vi "NUM TO 2D LED (SubVI).vi"(1 "A":dbl) -> (0 "transposed array":bool[][](array[boolean]))   [LabVIEW 2019]
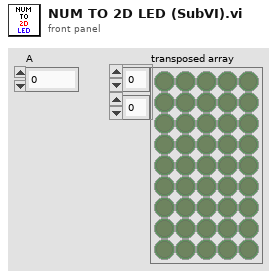
[diagram p1: front panel]
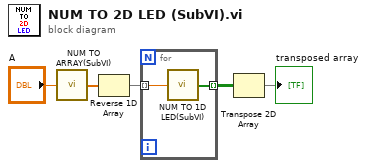
[diagram p0: block diagram]
diagram:
  n1 = call "NUM TO ARRAY(SubVI).vi"("A"="A") -> ("Array"=w2:dbl[])
  n2 = Reverse 1D Array(array=w2) -> (reversed array=w3:dbl[])
  n3 = for {
    tunnel: w3 -> [w7] mode=indexing
    tunnel: [w6] -> w4 mode=indexing
    n4 = call "NUM TO 1D LED(SubVI).vi"("A"=w7) -> ("Array"=w6:bool[])
  }
  n5 = Transpose 2D Array(2D array=w4) -> (transposed array=→"transposed array":bool[][])
